vi "filter channels by classification.vi"(8 "error in (no error)":errorcluster, 10 "channel classification":T1, 11 "channels in":refnum<class "TBM channel.lvclass">[](array[class])) -> (0 "error out":errorcluster, 3 "filtered channels out":refnum<class "TBM channel.lvclass">[](array[class]))   [LabVIEW 2014, in "Shared Memory configuration.lvclass"]
uses:
  Shared Memory configuration.lvclass
  <vilib>/NI/Tag Bus Module Framework/channel/TBM channel.lvclass
  <vilib>/NI/Tag Bus Module Framework/channel/channel classification.ctl
  <vilib>/NI/Tag Bus Module Framework/channel/TBM channel.lvclass/TBM channel.ctl
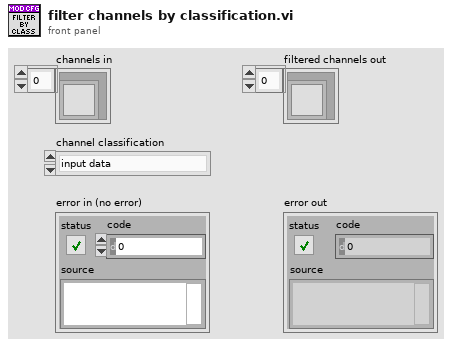
[diagram p1: front panel]
types:
  T1 = typedef "TBM channel.lvclass/channel classification.ctl" = enum16{"input data", "output data", "processing parameter", "processing result"}
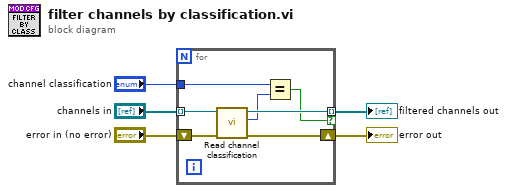
[diagram p0: block diagram]
diagram:
  n1 = for {
    shift-right: [w8] -> w1
    shift-left: "error in (no error)" -> [w12]
    tunnel: "channel classification" -> [w11]
    tunnel: "channels in" -> [w10] mode=indexing
    tunnel: [w9] -> w2 mode=indexing if=w6
    n2 = call <vilib>:"Read channel classification.vi"("error in"=w12, "channel in"=w10) -> ("error out"=w8:errorcluster, "channel classification"=w7:T1, "channel out"=w9:refnum<class "TBM channel.lvclass">)  [unwired: 7 in]
    n3 = Equal?(x=w11, y=w7) -> (x = y?=w6:bool)
  }
  "filtered channels out" <- w2
  "error out" <- w1
